vi "Request Single Measurement - Continuous Mode.vi"(0 "VISA resource name":refnum<visa-resource-name>, 7 "Single Measurement Type (Raw Accelerometer and Angular Rate)":u16(ring) items=["Raw Accelerometer and Angular Rate", "DeltaAngle & DeltaVelocity", "Orientation Matrix", "Orientation Update Matrix", "Acceleration, Angular Rate & Magnetometer Vectors", "Euler Angles", "Temperatures", "Gyro Stabilized Acceleration, Angular Rate & Magnetometer"], 11 "error in (no error)":errorcluster) -> (4 "VISA resource name out":refnum<visa-resource-name>, 15 "error out":errorcluster)   [LabVIEW 2012, in "MicroStrain 3DM-GXx.lvlib"]
doc: "Request a single measurement from the device during continuous measurement operation. The response from the device must be read and parsed using the Fetch Messages and Parse Message VIs ."
uses:
  <instrlib>/MicroStrain 3DM-GXx/MicroStrain 3DM-GXx.lvlib
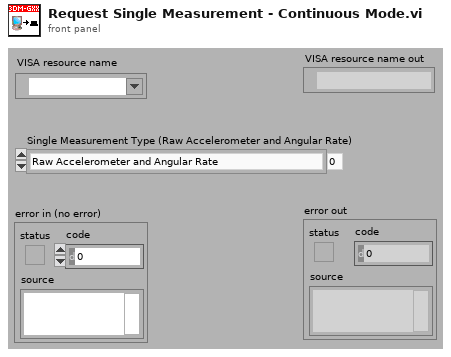
[diagram p1: front panel]
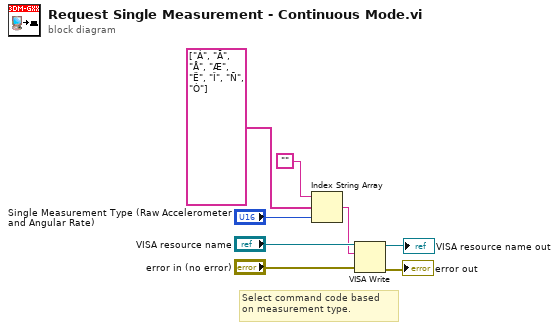
[diagram p0: block diagram]
diagram:
  # "Select command code based \non measurement type."
  n1 = Index String Array(1:"Single Measurement Type (Raw Accelerometer and Angular Rate)", 2:string[] ["Á", "Ã", "Å", "Æ", "Ë", "Î", "Ñ", "Ò"] ("string array"), 3:"" ("string (\"\")")) -> (0:w1:string)
  n2 = VISA Write(VISA resource name="VISA resource name", write buffer=w1, error in (no error)="error in (no error)") -> (VISA resource name out=→"VISA resource name out":refnum<visa-resource-name>, error out=→"error out":errorcluster)  [unwired: 1 out]
